vi "Apply Action.vi"(6 "Action":T1, 11 "VI Refnum":refnum<vi>) -> (0 "error out":errorcluster)   [LabVIEW 2015, in "Debugger.lvclass"]
uses:
  Debugger.lvclass
  Action.ctl
  <vilib>/Utility/miscctls.llb/LVRectTypeDef.ctl
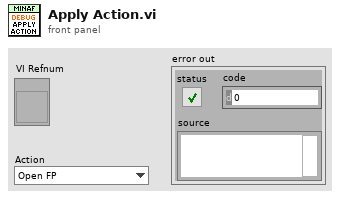
[diagram p1: front panel]
types:
  T1 = typedef "Debugger.lvclass/Action.ctl" = enum16{"Open FP", "Close FP", "Open BD", "Close BD", "Abort", "Enable Toolbar", "Move FP Up", "Move FP Down", "Move FP Left", "Move FP Right"}
  T2 = enum32{"Invalid", "Standard", "Closed", "Hidden", "Minimized", "Maximized"}
  T3 = typedef "LVRectTypeDef.ctl" = cluster{"Left":i16, "Top":i16, "Right":i16, "Bottom":i16}
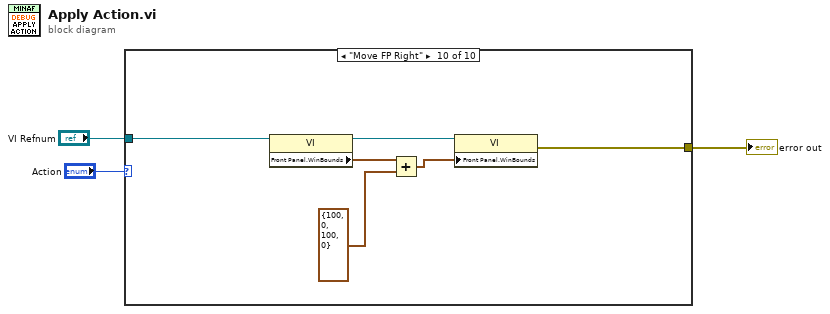
[diagram p0: block diagram]
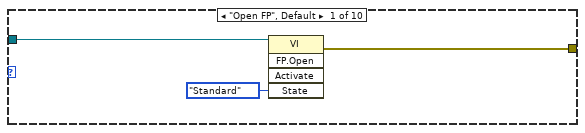
[diagram p2: hidden frame]
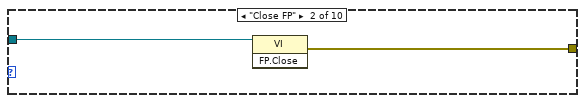
[diagram p3: hidden frame]
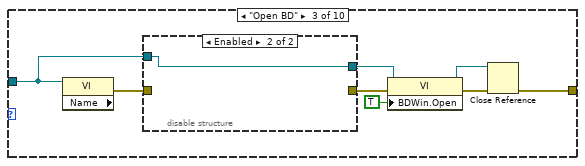
[diagram p4: hidden frame]
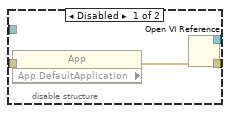
[diagram p5: hidden frame]
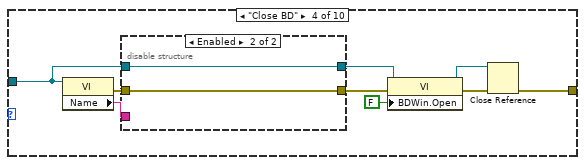
[diagram p6: hidden frame]
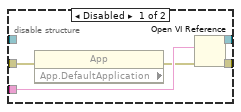
[diagram p7: hidden frame]
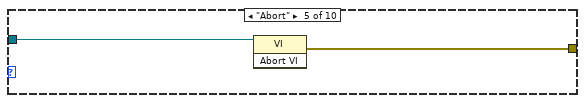
[diagram p8: hidden frame]
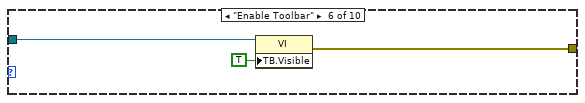
[diagram p9: hidden frame]
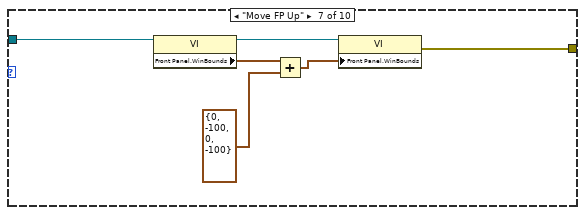
[diagram p10: hidden frame]
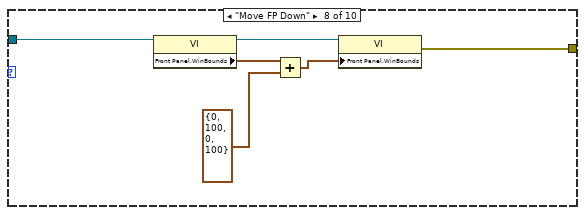
[diagram p11: hidden frame]
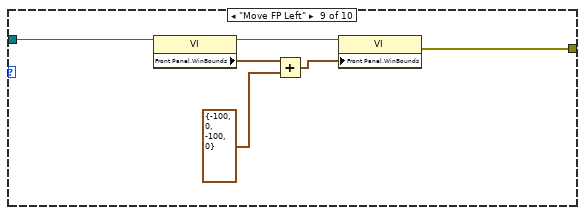
[diagram p12: hidden frame]
diagram:
  n1 = case shown="\"Move FP Right\"" "Action" {
    tunnel: "VI Refnum" -> [w6 w8 w9 w22 w39 w42 w47 w53 w59 w65]
    tunnel: [w4 w7 w11 w24 w38 w40 w48 w54 w60 w66] -> w1
    frame "Open FP", Default {
      n2 = invoke class="VI" method="FP.Open"(reference=w6, "State"=T2."Standard") -> (error out=w4:errorcluster)  [unwired: 3 in, 4 out]
    }
    frame "Close FP" {
      n3 = invoke class="VI" method="FP.Close"(reference=w8) -> (error out=w7:errorcluster)  [unwired: 2 in, 2 out]
    }
    frame "Open BD" {
      n4 = property class="VI" props=["Name"](reference=w9) -> (error out=w14:errorcluster)  [unwired: 1 in, 2 out]
      n5 = disable-structure shown="Enabled" {
        disable-tunnel: [w20 w21] -> w15
        disable-tunnel: w14 -> [w19 _]
        disable-tunnel: [w17 _] -> w13
        disable-tunnel: w9 -> [_ w21]
        frame Disabled {
          n6 = property class="App" props=["App.DefaultApplication"](error in=w19) -> (error out=w18:errorcluster)  [unwired: 1 in, 2 out]
          n7 = Open VI Reference(error in (no error)=w18) -> (vi reference=w20:refnum<vi>, error out=w17:errorcluster)  [unwired: 1 in, 4 out]
        }
        frame Enabled {
        }
      }
      n8 = property class="VI"(reference=w15, error in=w13, "BDWin.Open"=TRUE ("Block Diagram Window:Open")) -> (reference out=w10:refnum<vi>, error out=w12:errorcluster)
      n9 = Close Reference(reference=w10, error in (no error)=w12) -> (error out=w11:errorcluster)
    }
    frame "Close BD" {
      n10 = property class="VI"(reference=w22) -> (error out=w27:errorcluster, "Name"=w30:string)  [unwired: 1 in, 1 out]
      n11 = disable-structure shown="Enabled" {
        disable-tunnel: w30 -> [w35 _]
        disable-tunnel: [w34 w37] -> w28
        disable-tunnel: w27 -> [w33 w36]
        disable-tunnel: [w31 w36] -> w26
        disable-tunnel: w22 -> [_ w37]
        frame Disabled {
          n12 = property class="App" props=["App.DefaultApplication"](error in=w33) -> (error out=w32:errorcluster)  [unwired: 1 in, 2 out]
          n13 = Open VI Reference(vi path=w35, error in (no error)=w32) -> (vi reference=w34:refnum<vi>, error out=w31:errorcluster)  [unwired: 4 out]
        }
        frame Enabled {
        }
      }
      n14 = property class="VI"(reference=w28, error in=w26, "BDWin.Open"=FALSE ("Block Diagram Window:Open")) -> (reference out=w23:refnum<vi>, error out=w25:errorcluster)
      n15 = Close Reference(reference=w23, error in (no error)=w25) -> (error out=w24:errorcluster)
    }
    frame "Abort" {
      n16 = invoke class="VI" method="Abort VI"(reference=w39) -> (error out=w38:errorcluster)  [unwired: 2 in, 2 out]
    }
    frame "Enable Toolbar" {
      n17 = property class="VI"(reference=w42, "TB.Visible"=TRUE ("Tool Bar:Visible")) -> (error out=w40:errorcluster)  [unwired: 1 in, 1 out]
    }
    frame "Move FP Up" {
      n18 = property class="VI"(reference=w47) -> (reference out=w46:refnum<vi>, "Front Panel.WinBounds"=w45:T3)  [unwired: 1 in, 1 out]
      n19 = Add(x=w45, y=T3 {"Left"=0, "Top"=-100, "Right"=0, "Bottom"=-100}) -> (x+y=w44:T3)
      n20 = property class="VI"(reference=w46, "Front Panel.WinBounds"=w44) -> (error out=w48:errorcluster)  [unwired: 1 in, 1 out]
    }
    frame "Move FP Down" {
      n21 = property class="VI"(reference=w53) -> (reference out=w52:refnum<vi>, "Front Panel.WinBounds"=w51:T3)  [unwired: 1 in, 1 out]
      n22 = Add(x=w51, y=T3 {"Left"=0, "Top"=100, "Right"=0, "Bottom"=100}) -> (x+y=w50:T3)
      n23 = property class="VI"(reference=w52, "Front Panel.WinBounds"=w50) -> (error out=w54:errorcluster)  [unwired: 1 in, 1 out]
    }
    frame "Move FP Left" {
      n24 = property class="VI"(reference=w59) -> (reference out=w58:refnum<vi>, "Front Panel.WinBounds"=w57:T3)  [unwired: 1 in, 1 out]
      n25 = Add(x=w57, y=T3 {"Left"=-100, "Top"=0, "Right"=-100, "Bottom"=0}) -> (x+y=w56:T3)
      n26 = property class="VI"(reference=w58, "Front Panel.WinBounds"=w56) -> (error out=w60:errorcluster)  [unwired: 1 in, 1 out]
    }
    frame "Move FP Right" {
      n27 = property class="VI"(reference=w65) -> (reference out=w64:refnum<vi>, "Front Panel.WinBounds"=w63:T3)  [unwired: 1 in, 1 out]
      n28 = Add(x=w63, y=T3 {"Left"=100, "Top"=0, "Right"=100, "Bottom"=0}) -> (x+y=w62:T3)
      n29 = property class="VI"(reference=w64, "Front Panel.WinBounds"=w62) -> (error out=w66:errorcluster)  [unwired: 1 in, 1 out]
    }
  }
  "error out" <- w1
